vi "Run.vi"(8 "error in (no error)":errorcluster, 9 "Time Ratio used":dbl, 10 "Maze (0: Empty, -1: Enemy. >0: Teammate":i32[][](array[numeric]), 11 "Line Dancer in":refnum<class "Line Dancer.lvclass">) -> (0 "error out":errorcluster, 1 "Direction":T1, 2 "Action":T2, 3 "Line Dancer out":refnum<class "Line Dancer.lvclass">, 4 "Replicated":refnum<class "Runner.lvclass">)   [LabVIEW 2014, in "Line Dancer.lvclass"]
uses:
  Line Dancer.lvclass
  Action Enum.ctl
  Direction Enum.ctl
  Runner.lvclass
  Line Dancer.lvclass/Line Dancer.ctl
  Line Dancer Type.ctl
  SquareBattle.lvclass
  Formics/Formics.lvclass
panel:
  # "NOTICE - YOU MUST NOT REMOVE THIS NOTICE. PER THE FOLLOWING LICENSE, YOU MAY REPRODUCE THIS SOFTWARE PROVIDED YOU FOLLOW THE TERMS\nOF THE LICENSE.\n\n---BEGIN BSD LICENSE (http://opensource.org/licenses/BSD-2-Clause)---\nCopyright (c) 2015, Endigit, Inc. <robert@endigit.com>\nAll rights reserved.\n\nRedistribution and use in source and binary forms, with or without modification, are permitted provided that the following conditions are met:\n\n1. Redistributions of source code must retain the above copyright notice, this list of conditions and the following disclaimer.\n\n2. Redistributions in binary form must reproduce the above copyright notice, this list of conditions and the following disclaimer in the documentation and/or other \nmaterials provided with the distribution.\n\nTHIS SOFTWARE IS PROVIDED BY THE COPYRIGHT HOLDERS AND CONTRIBUTORS \"AS IS\" AND ANY EXPRESS OR IMPLIED WARRANTIES, INCLUDING, BUT NOT \nLIMITED TO, THE IMPLIED WARRANTIES OF MERCHANTABILITY AND FITNESS FOR A PARTICULAR PURPOSE ARE DISCLAIMED. IN NO EVENT SHALL THE COPYRIGHT \nHOLDER OR CONTRIBUTORS BE LIABLE FOR ANY DIRECT, INDIRECT, INCIDENTAL, SPECIAL, EXEMPLARY, OR CONSEQUENTIAL DAMAGES (INCLUDING, BUT NOT \nLIMITED TO, PROCUREMENT OF SUBSTITUTE GOODS OR SERVICES; LOSS OF USE, DATA, OR PROFITS; OR BUSINESS INTERRUPTION) HOWEVER CAUSED AND ON \nANY THEORY OF LIABILITY, WHETHER IN CONTRACT, STRICT LIABILITY, OR TORT (INCLUDING NEGLIGENCE OR OTHERWISE) ARISING IN ANY WAY OUT OF THE USE \nOF THIS SOFTWARE, EVEN IF ADVISED OF THE POSSIBILITY OF SUCH DAMAGE.\n---END BSD LICENSE---"
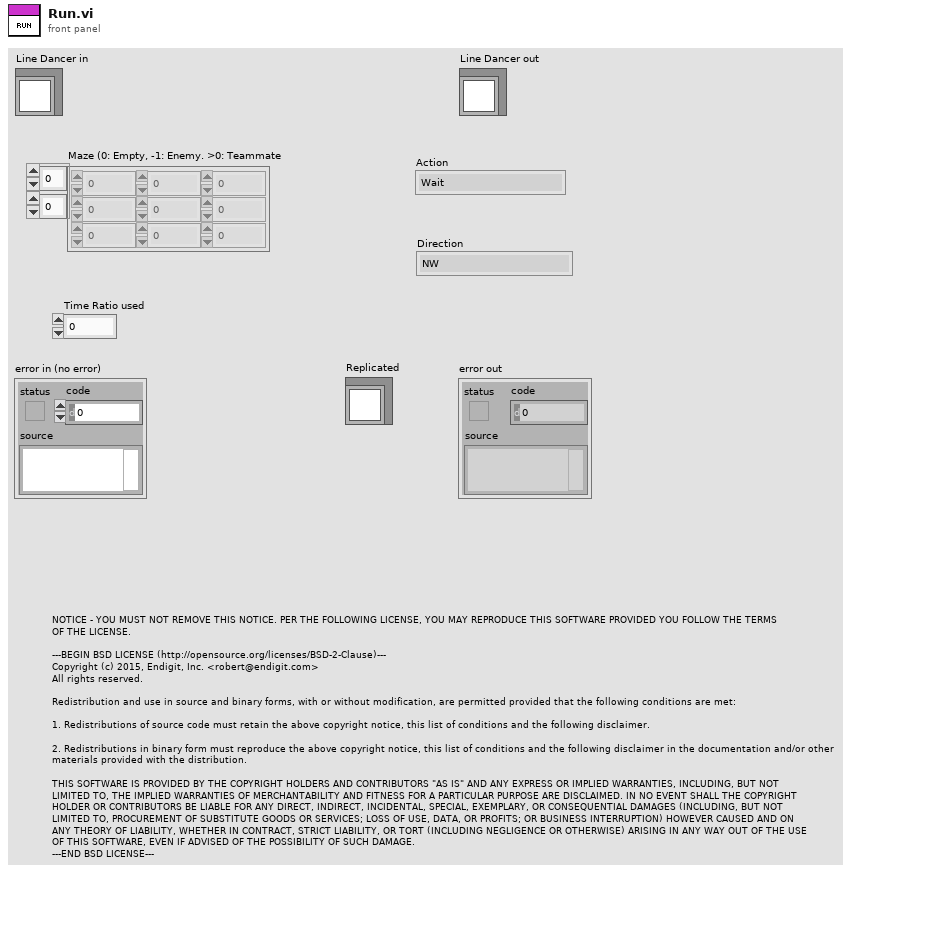
[diagram p1: front panel]
types:
  T1 = typedef "SquareBattle.lvclass/Direction Enum.ctl" = enum16{"NW", "N", "NE", "E", "SE", "S", "SW", "W"}
  T2 = typedef "SquareBattle.lvclass/Action Enum.ctl" = enum16{"Wait", "Move", "Attack", "Replicate"}
  T3 = typedef "Line Dancer.lvclass/Line Dancer Type.ctl" = enum16{"Top", "Bottom", "Start"}
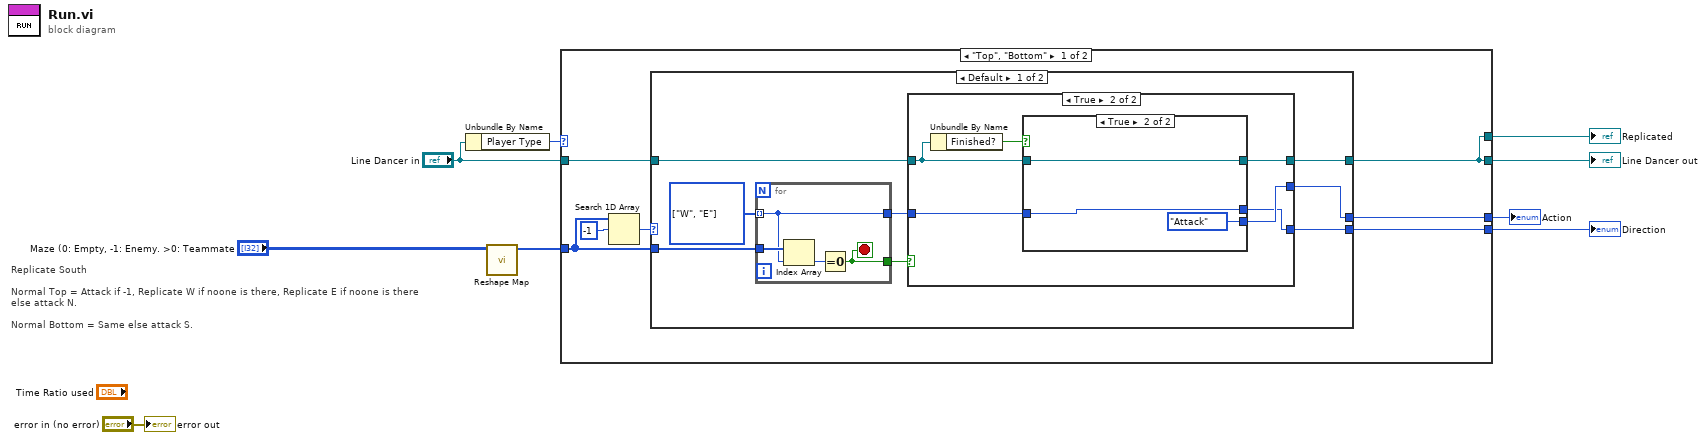
[diagram p0: block diagram]
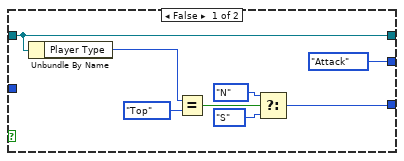
[diagram p2: hidden frame]
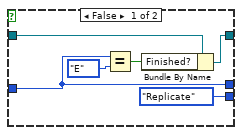
[diagram p3: hidden frame]
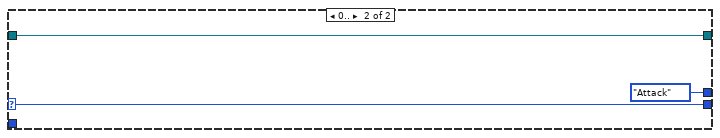
[diagram p4: hidden frame]
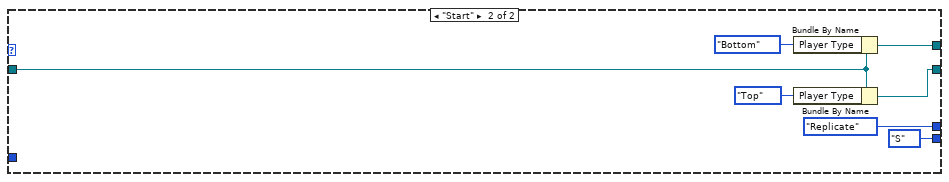
[diagram p5: hidden frame]
diagram:
  # "Replicate South\n\nNormal Top = Attack if -1, Replicate W if noone is there, Replicate E if noone is there\nelse attack N.\n\nNormal Bottom = Same else attack S."
  n1 = Unbundle By Name("Line Dancer in") -> ("Player Type"=w4:T3)
  n2 = call "Reshape Map.vi"("Maze (0: Empty, -1: Enemy. >0: Teammate"="Maze (0: Empty, -1: Enemy. >0: Teammate") -> ("Map"=w5:i32[])  [unwired: 9 in, 1 out]
  n3 = case shown="\"Top\", \"Bottom\"" w4 {
    tunnel: [w14 Action_Enum."Replicate" ("Action")] -> w8
    tunnel: [w13 Direction_Enum."S" ("Direction")] -> w7
    tunnel: w5 -> [w12 _]
    tunnel: [w10 w58] -> w3
    tunnel: [w10 w57] -> w2
    tunnel: "Line Dancer in" -> [w11 w55]
    frame "Top", "Bottom" {
      n4 = Search 1D Array(1D array=w12, element=-1) -> (index of element=w15:i32)  [unwired: 1 in]
      n5 = case shown="Default" w15 {
        selector: w15 -> [_ w53]
        tunnel: [w21 Action_Enum."Attack" ("Action")] -> w14
        tunnel: [w19 w53] -> w13
        tunnel: w12 -> [w24 _]
        tunnel: [w17 w52] -> w10
        tunnel: w11 -> [w18 w52]
        frame Default {
          w23 = T1[] [enum."W", enum."E"] items=["NW", "N", "NE", "E", "SE", "S", "SW", "W"]
          n6 = for {
            tunnel: w24 -> [w51]
            tunnel: w23 -> [w50] mode=indexing
            tunnel: [w50] -> w20
            tunnel: [w48] -> w22
            stop <- w48 stop-if-true
            n7 = Index Array(array=w51, index=w50) -> (element=w49:i32)
            n8 = Equal To 0?(x=w49) -> (x = 0?=w48:bool)
          }
          n9 = case shown="True" w22 {
            tunnel: [Action_Enum."Attack" ("Action") w38] -> w21
            tunnel: [w27 w36] -> w19
            tunnel: w20 -> [_ w37]
            tunnel: w18 -> [w31 w34]
            tunnel: [w31 w33] -> w17
            frame False {
              n10 = Unbundle By Name(w31) -> ("Player Type"=w30:T3)
              n11 = Equal?(x=w30, y=Line_Dancer_Type."Top") -> (x = y?=w28:bool)
              n12 = Select(t=Direction_Enum."N" ("Direction"), s=w28, f=Direction_Enum."S" ("Direction")) -> (s? t:f=w27:T1)
            }
            frame True {
              n13 = Unbundle By Name(w34) -> ("Finished?"=w35:bool)
              n14 = case shown="True" w35 {
                tunnel: [Action_Enum."Replicate" ("f") Action_Enum."Attack" ("f")] -> w38
                tunnel: w37 -> [w43 w45]
                tunnel: [w43 w45] -> w36
                tunnel: w34 -> [w41 w46]
                tunnel: [w39 w46] -> w33
                frame False {
                  n15 = Equal?(x=w43, y=Direction_Enum."E") -> (x = y?=w40:bool)
                  n16 = Bundle By Name(cluster=w41, "Finished?"=w40) -> (w39:refnum<class "Line Dancer.lvclass">)
                }
                frame True {
                }
              }
            }
          }
        }
        frame 0.. {
        }
      }
    }
    frame "Start" {
      n17 = Bundle By Name(cluster=w55, "Player Type"=Line_Dancer_Type."Bottom") -> (w58:refnum<class "Line Dancer.lvclass">)
      n18 = Bundle By Name(cluster=w55, "Player Type"=Line_Dancer_Type."Top") -> (w57:refnum<class "Line Dancer.lvclass">)
    }
  }
  "Line Dancer out" <- w2
  "Action" <- w8
  "Direction" <- w7
  "Replicated" <- w3
  "error out" <- "error in (no error)"
